vi "XLP80_Action_InitGlobals.vi"(8 "err in":errorcluster) -> (0 "err out":errorcluster)   [LabVIEW 2021]
uses:
  XLP80_State_V001.llb/XLP80_State_TDefEnumGlobalState.ctl
  XLP80_State_V001.llb/XLP80_State_TDefEnumStateDatalog.ctl
  XLP80_CAN/1886_PEAK_TDefEnumCANState.ctl
  XLP80_General_Libs/WL_Libs_V14.25/WL_Frontpanel_V14.01.llb/WL_Frontpanel_GblStatus.vi
  XLP80_Globals/XLP80_Globals_Status.vi
  XLP80_Globals/XLP80_Globals_Action.vi
  XLP80_State_V001.llb/XLP80_State_Globals.vi
  XLP80_General_Libs/WL_Libs_V14.25/WL_Profile_V14.00.llb/WL_Profile_Globals.vi
  XLP80_Globals/XLP80_CAN_Globals.vi
  FCE_TS_SMART_V001.llb/XLP80_SMART_GUIGlobals.vi
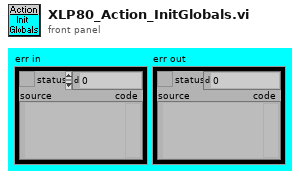
[diagram p1: front panel]
types:
  T1 = typedef "1886_PEAK_TDefEnumCANState.ctl" = enum16{"Wait Start", "Start CAN", "Run CAN", "Stop CAN"}
  T2 = typedef "XLP80_State_TDefEnumStateDatalog.ctl" = enum16{"default", "StartLog", "Log", "StopLog", "NewFile"}
  T3 = typedef "XLP80_State_TDefEnumGlobalState.ctl" = enum16{"HV & Software", "Basis Funktion", "Power Management", "Operational Mode", "Shutdown", "Alarm"}
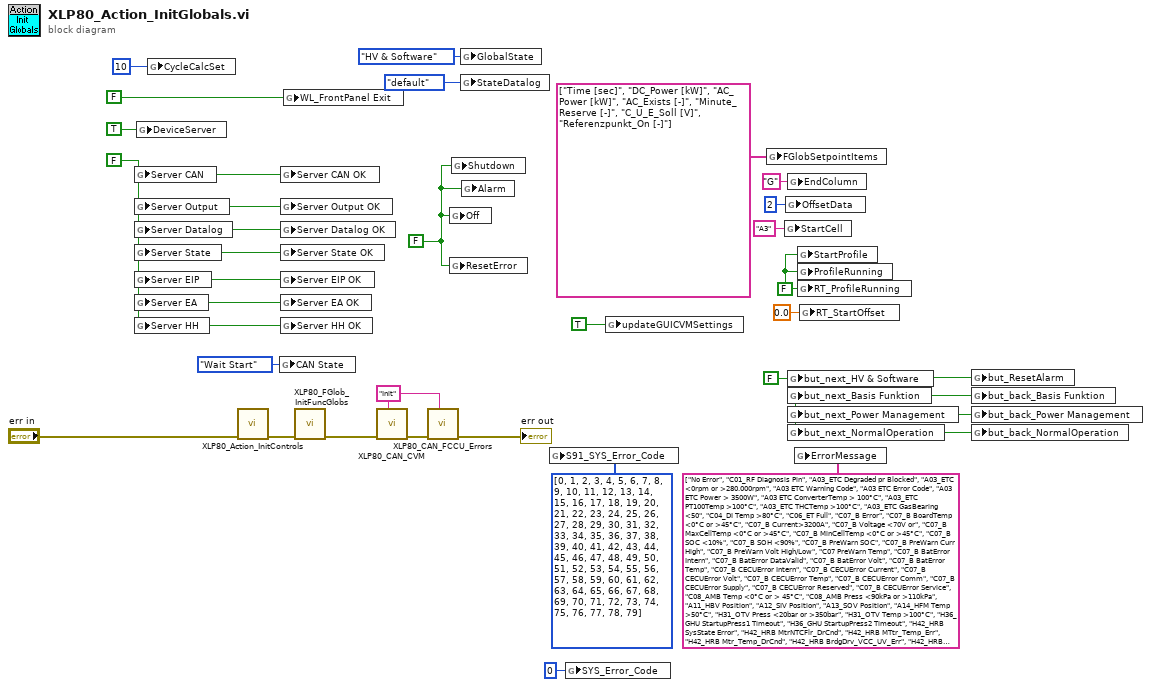
[diagram p0: block diagram]
diagram:
  w1 = "Init" ("Function")
  w3 = FALSE ("but_next_HV & Software")
  w14 = FALSE ("RT_ProfileRunning")
  w4 = FALSE ("Purge_Man")
  w9 = FALSE ("Server Alarm")
  n1 = global write "XLP80_Globals_Action.vi" "Server CAN"(w9) -> ()
  n2 = global write "XLP80_Globals_Action.vi" "Server Output"(w9) -> ()
  n3 = global write "XLP80_Globals_Action.vi" "Server Datalog"(w9) -> ()
  n4 = global write "XLP80_Globals_Action.vi" "Server State"(w9) -> ()
  n5 = global write "XLP80_Globals_Action.vi" "Server EIP"(w9) -> ()
  n6 = global write "XLP80_Globals_Action.vi" "Server EA"(w9) -> ()
  n7 = global write "XLP80_Globals_Action.vi" "Server HH"(w9) -> ()
  n8 = global write "XLP80_Globals_Status.vi" "DeviceServer"(TRUE ("DeviceServer")) -> ()
  n9 = global write "XLP80_Globals_Action.vi" "CycleCalcSet"(u32 10 ("CycleCalcSet")) -> ()
  n10 = call "XLP80_Action_InitControls.vi"("err in"="err in") -> ("err out"=w23:errorcluster)  [unwired: 10 in]
  n11 = global write "XLP80_CAN_Globals.vi" "CAN State"(1886_PEAK_TDefEnumCANState."Wait Start" ("CAN State")) -> ()
  n12 = global write "XLP80_Globals_Action.vi" "Server CAN OK"(w9) -> ()
  n13 = global write "XLP80_Globals_Action.vi" "Server Output OK"(w9) -> ()
  n14 = global write "XLP80_Globals_Action.vi" "Server Datalog OK"(w9) -> ()
  n15 = global write "XLP80_Globals_Action.vi" "Server State OK"(w9) -> ()
  n16 = global write "XLP80_Globals_Action.vi" "Server EIP OK"(w9) -> ()
  n17 = global write "XLP80_Globals_Action.vi" "Server EA OK"(w9) -> ()
  n18 = global write "XLP80_Globals_Action.vi" "Server HH OK"(w9) -> ()
  n19 = global write "WL_Frontpanel_GblStatus.vi" "WL_FrontPanel Exit"(FALSE ("BL_FrontPanel Exit")) -> ()
  n20 = call "XLP80_FGlob_InitFuncGlobs.vi"("err in"=w23) -> ("err out"=w11:errorcluster)  [unwired: 10 in]
  n21 = call "XLP80_CAN_CVM.vi"("Function"=w1, "err in"=w11) -> ("err out"=w10:errorcluster)  [unwired: 9 in]
  n22 = call "XLP80_CAN_FCCU_Errors.vi"("Function"=w1, "err in"=w10) -> ("err out"=→"err out":errorcluster)  [unwired: 7 in, 2 out]
  n23 = global write "XLP80_Globals_Action.vi" "Off"(w4) -> ()
  n24 = global write "XLP80_Globals_Action.vi" "ResetError"(w4) -> ()
  n25 = global write "XLP80_Globals_Action.vi" "Shutdown"(w4) -> ()
  n26 = global write "XLP80_State_Globals.vi" "GlobalState"(XLP80_State_TDefEnumGlobalState."HV & Software" ("GlobalState")) -> ()
  n27 = global write "XLP80_State_Globals.vi" "StateDatalog"(XLP80_State_TDefEnumStateDatalog."default" ("StateDatalog")) -> ()
  n28 = global write "XLP80_Globals_Action.vi" "Alarm"(w4) -> ()
  n29 = global write "XLP80_Globals_Status.vi" "S91_SYS_Error_Code"(u32[] [0, 1, 2, 3, 4, 5, 6, 7, 8, 9, 10, 11, 12, 13, 14, 15, 16, 17, 18, 19, 20, 21, 22, 23, 24, 25, 26, 27, 28, 29, 30, 31, 32, 33, 34, 35, 36, 37, 38, 39, 40, 41, 42, 43, 44, 45, 46, 47, 48, 49, 50, 51, 52, 53, 54, 55, 56, 57, 58, 59, 60, 61, 62, 63, 64, 65, 66, 67, 68, 69, 70, 71, 72, 73, 74, 75, 76, 77, 78, 79] ("S91_SYS_Error_Code")) -> ()
  n30 = global write "XLP80_Globals_Status.vi" "SYS_Error_Code"(u32 0 ("SYS_Error_Code")) -> ()
  n31 = global write "XLP80_SMART_GUIGlobals.vi" "updateGUICVMSettings"(TRUE ("updateSettings")) -> ()
  n32 = global write "WL_Profile_Globals.vi" "FGlobSetpointItems"(string[] ["Time [sec]", "DC_Power [kW]", "AC_Power [kW]", "AC_Exists [-]", "Minute_Reserve [-]", "C_U_E_Soll [V]", "Referenzpunkt_On [-]"] ("FGlobSetpointItems")) -> ()
  n33 = global write "WL_Profile_Globals.vi" "StartCell"("A3" ("StartCell")) -> ()
  n34 = global write "WL_Profile_Globals.vi" "OffsetData"(2 ("OffsetData")) -> ()
  n35 = global write "WL_Profile_Globals.vi" "EndColumn"("G" ("EndColumn")) -> ()
  n36 = global write "XLP80_Globals_Action.vi" "but_next_HV & Software"(w3) -> ()
  n37 = global write "XLP80_Globals_Action.vi" "but_next_Basis Funktion"(w3) -> ()
  n38 = global write "XLP80_Globals_Action.vi" "but_next_Power Management"(w3) -> ()
  n39 = global write "XLP80_Globals_Action.vi" "but_next_NormalOperation"(w3) -> ()
  n40 = global write "XLP80_Globals_Status.vi" "ErrorMessage"(string[] ["No Error", "C01_RF Diagnosis Pin", "A03_ETC Degraded pr Blocked", "A03_ETC <0rpm or >280.000rpm", "A03 ETC Warning Code", "A03 ETC Error Code", "A03 ETC Power > 3500W", "A03 ETC ConverterTemp > 100°C", "A03_ETC PT100Temp >100°C", "A03_ETC THCTemp >100°C", "A03_ETC GasBearing <50", "C04_DI Temp >80°C", "C06_ET Full", "C07_B Error", "C07_B BoardTemp <0°C or >45°C", "C07_B Current>3200A", "C07_B Voltage <70V or", "C07_B MaxCellTemp <0°C or >45°C", "C07_B MinCellTemp <0°C or >45°C", "C07_B SOC <10%", "C07_B SOH <90%", "C07_B PreWarn SOC", "C07_B PreWarn Curr High", "C07_B PreWarn Volt High/Low", "C07 PreWarn Temp", "C07_B BatError Intern", "C07_B BatError DataValid", "C07_B BatError Volt", "C07_B BatError Temp", "C07_B CECUError Intern", "C07_B CECUError Current", "C07_B CECUError Volt", "C07_B CECUError Temp", "C07_B CECUError Comm", "C07_B CECUError Supply", "C07_B CECUError Reserved", "C07_B CECUError Service", "C08_AMB Temp <0°C or > 45°C", "C08_AMB Press <90kPa or >110kPa", "A11_HBV Position", "A12_SIV Position", "A13_SOV Position", "A14_HFM Temp >50°C", "H31_OTV Press <20bar or >350bar", "H31_OTV Temp >100°C", "H36_GHU StartupPress1 Timeout", "H36_GHU StartupPress2 Timeout", "H42_HRB SysState Error", "H42_HRB MtrNTCFlr_DrCnd", "H42_HRB MTtr_Temp_Err", "H42_HRB Mtr_Temp_DrCnd", "H42_HRB BrdgDrv_VCC_UV_Err", "H42_HRB ShortToGround_Err", "H42_HRB ShortToBat_Err", "H42_HRB E2E_Err", "H42_HRB SpdLimitRq_Err", "H42_HRB Blocked_Err", "H42_HRBBatt_Vltg_Err", "H42_HRB ECU_Temp_Err", "H42_HRB ECU_Temp_DrCnd", "H42_HRB KNF Error", "H42_WT Tank Full", "H51_STK LowCellVolt <200mV", "H51_STK TotalVolt <31V or >75V", "H51_STK Startup CellVolt Timeout", "H51_STK Shutdown CellVolt Timeout", "H53_PV Startup Timeout", "C54_SI Temp >80°C", "H55_SI Press >2,5bar", "H62_HLD ErrorCode = 3", "H62_HLD Concentration >122.500ppm", "H63_HLD ErrorCode = 3", "H63_HLD Concentration >122.500ppm", "E71_DCDC Precharge", "E71_DCDC Operational", "E74_ISO R <0kOhm", "E74_ISO IsoError", "E74_ISO Err Chassis", "E74_ISO Sysstoer", "E74_ISO IsoWarn"] ("ErrorMessage")) -> ()
  n41 = global write "WL_Profile_Globals.vi" "StartProfile"(w14) -> ()
  n42 = global write "WL_Profile_Globals.vi" "ProfileRunning"(w14) -> ()
  n43 = global write "WL_Profile_Globals.vi" "RT_ProfileRunning"(w14) -> ()
  n44 = global write "WL_Profile_Globals.vi" "RT_StartOffset"(sgl 0.0 ("RT_StartOffset")) -> ()
  n45 = global write "XLP80_Globals_Action.vi" "but_ResetAlarm"(w3) -> ()
  n46 = global write "XLP80_Globals_Action.vi" "but_back_Basis Funktion"(w3) -> ()
  n47 = global write "XLP80_Globals_Action.vi" "but_back_Power Management"(w3) -> ()
  n48 = global write "XLP80_Globals_Action.vi" "but_back_NormalOperation"(w3) -> ()
